vi "init.vi"(8 "error in (no error)":errorcluster, 11 "_cameraBase in":refnum<class "_cameraBase.lvclass">) -> (0 "error out":errorcluster, 3 "_cameraBase out":refnum<class "_cameraBase.lvclass">)   [LabVIEW 2018, in "_cameraBase.lvclass"]
uses:
  _cameraBase.lvclass
panel:
  in  "resource name out":string
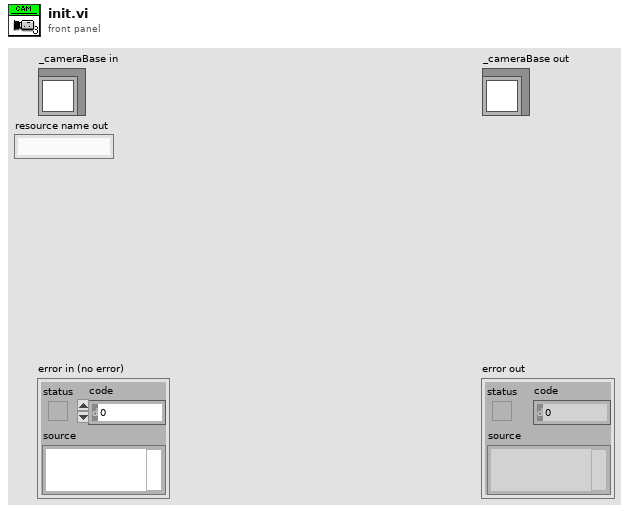
[diagram p1: front panel]
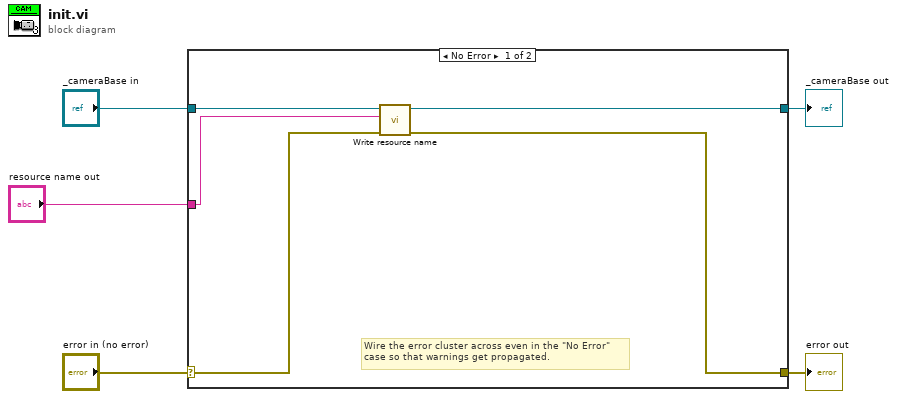
[diagram p0: block diagram]
diagram:
  n1 = case shown="No Error" "error in (no error)" {
    selector: "error in (no error)" -> [w8 w12]
    tunnel: [w7 w12] -> w4
    tunnel: [w9 w11] -> w2
    tunnel: "_cameraBase in" -> [w10 w11]
    tunnel: "resource name out" -> [w6 _]
    frame No Error {
      # "Wire the error cluster across even in the \"No Error\"\ncase so that warnings get propagated."
      n2 = call-dynamic "Write resource name.vi"("error in (no error)"=w8, "resource name"=w6, "_cameraBase in"=w10) -> ("error out"=w7:errorcluster, "_cameraBase out"=w9:refnum<class "_cameraBase.lvclass">)  [unwired: 7 in]
    }
    frame Error {
    }
  }
  "error out" <- w4
  "_cameraBase out" <- w2
